vi "Is Resource Available.vi"(9 "Data":string, 11 "WebSocket Client in":refnum<class "WebSocket Client.lvclass">) -> (0 "Is Service Available":bool, 1 "Data Out":string, 3 "WebSocket Client out":refnum<class "WebSocket Client.lvclass">)   [LabVIEW 2016, in "WebSocket Actors.lvlib" / "WebSocket Client.lvclass"]
uses:
  WebSocket Client.lvclass
  WebSocket Server/WebSocket Server.lvclass
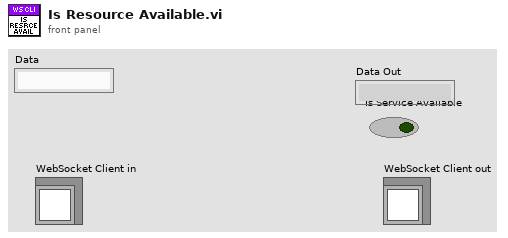
[diagram p1: front panel]
types:
  T1 = typedef "WebSocket Actors.lvlib/WebSocket Server.lvclass/Http Response Codes.ctl" = u16
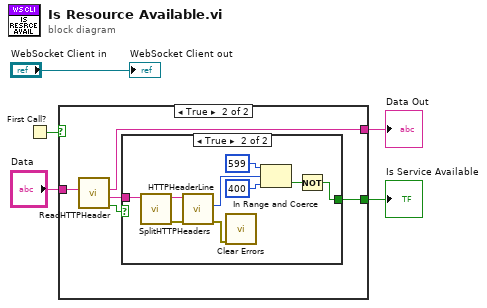
[diagram p0: block diagram]
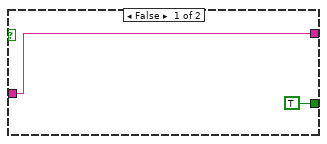
[diagram p2: hidden frame]
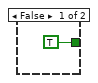
[diagram p3: hidden frame]
diagram:
  n1 = First Call?() -> (First Call?: T/F=w5:bool)
  n2 = case shown="True" w5 {
    tunnel: [w6 w11] -> w3
    tunnel: "Data" -> [w6 w12]
    tunnel: [TRUE w9] -> w2
    frame False {
    }
    frame True {
      n3 = call "ReadHTTPHeader.vi"("Data"=w12) -> ("Header Found"=w8:bool, "HTTP Header"=w10:string, "Data Out"=w11:string)  [unwired: 8 in]
      n4 = case shown="True" w8 {
        tunnel: w10 -> [_ w22]
        tunnel: [TRUE w15] -> w9
        frame False {
        }
        frame True {
          n5 = call "SplitHTTPHeaders.vi"("HTTP Header String"=w22) -> ("error out"=w20:errorcluster, "HTTP Request"=w21:string)  [unwired: 8 in, 1 out]
          n6 = call "HTTPHeaderLine.vi"("error in (no error)"=w20, "HTTP Request Line"=w21) -> ("error out"=w14:errorcluster, "Status Code"=w19:T1)  [unwired: 6 in, 2 out]
          n7 = call <vilib>:"Clear Errors.vi"("error in (no error)"=w14) -> ()  [unwired: 5 in, 2 out]
          n8 = In Range and Coerce(upper limit=u16 599, x=w19, lower limit=u16 400) -> (In Range?=w16:bool)  [unwired: 1 out]
          n9 = Not(x=w16) -> (.not. x?=w15:bool)
        }
      }
    }
  }
  "Is Service Available" <- w2
  "Data Out" <- w3
  "WebSocket Client out" <- "WebSocket Client in"
